vi "ICM Select Channel Names.vi"(10 "Enabled":bool[](array[boolean]), 11 "Channels":string[](array[string])) -> (3 "Enabled Channels":string[](array[string]))   [LabVIEW 2024]
doc: "ICM Select Channel Names.vi\n\nThis VI returns the names of the Channels that have been enabled in the configuration.\n\nInstrument Communication Module Version 1.0\nSeptember, 2017 Original Code Consulting David Thomson\n www.originalcode.com"
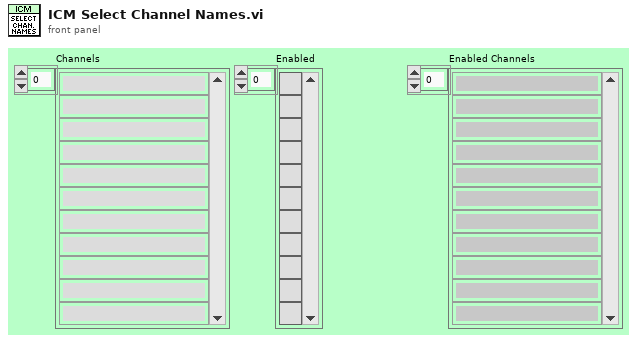
[diagram p1: front panel]
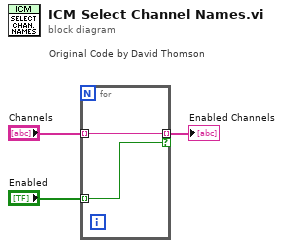
[diagram p0: block diagram]
diagram:
  n1 = for "Original Code by David Thomson" {
    tunnel: [w5] -> w1 mode=indexing if=w4
    tunnel: "Channels" -> [w5] mode=indexing
    tunnel: "Enabled" -> [w4] mode=indexing
  }
  "Enabled Channels" <- w1
